vi "Destroy multiple mailboxes.vi"(8 "error in (no error)":errorcluster, 10 "force destroy? (F)":bool, 11 "Mailboxes":T1[](array[typedef])) -> (0 "error out":errorcluster, 2 "Remaining elements":variant[][](array[variant]), 3 "Destroyed mailboxes":string[](array[string]))   [LabVIEW 2024, in "MessengerLib.lvlib"]
uses:
  MessengerLib.lvlib
  Data types/Mailbox address.ctl
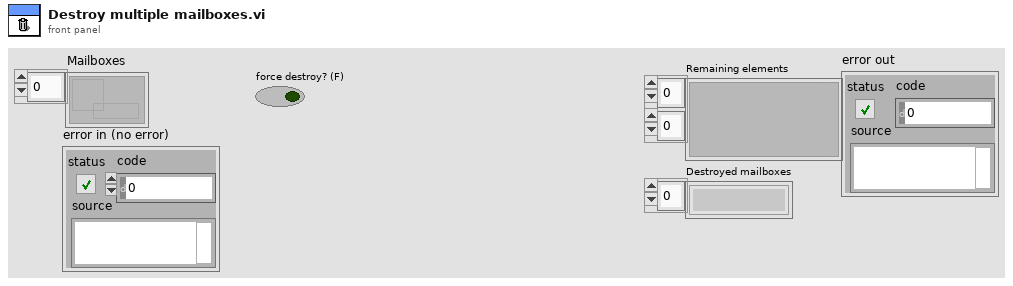
[diagram p1: front panel]
types:
  T1 = typedef "MessengerLib.lvlib/Mailbox address.ctl" = refnum<queue>
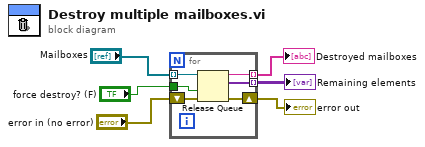
[diagram p0: block diagram]
diagram:
  n1 = for {
    tunnel: "Mailboxes" -> [w12] mode=indexing
    tunnel: [w10] -> w4 mode=indexing
    tunnel: [w9] -> w3 mode=indexing
    shift-right: [w8] -> w2
    shift-left: "error in (no error)" -> [w11]
    tunnel: "force destroy? (F)" -> [w7]
    n2 = Release Queue(queue=w12, force destroy? (F)=w7, error in (no error)=w11) -> (queue name=w9:string, remaining elements=w10:variant[], error out=w8:errorcluster)
  }
  "Remaining elements" <- w4
  "Destroyed mailboxes" <- w3
  "error out" <- w2
